vi "ImportBitmap2.vi"(8 "error in (no error)":errorcluster) -> (0 "error out":errorcluster, 1 "color table":u32[](array[colorbox]), 2 "pixmap data":u8[](array[numeric]), 3 "rect":T1, 5 "bit depth(8)":i32=8)   [LabVIEW 2013, in "main.lvlib"]
uses:
  main.lvlib
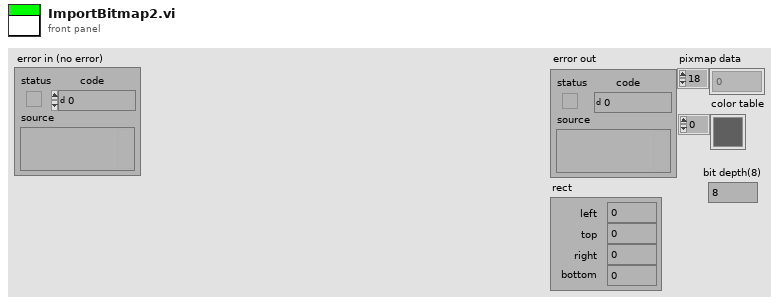
[diagram p1: front panel]
types:
  T1 = cluster{"left":i16, "top":i16, "right":i16, "bottom":i16}
  T2 = typedef "CLIP Refnum.ctl" = refnum<k1>
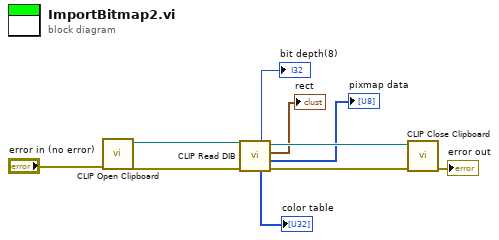
[diagram p0: block diagram]
diagram:
  n1 = call "CLIP Open Clipboard.vi"("error in (no error)"="error in (no error)") -> ("error out"=w9:errorcluster, "clipboard ref"=w10:T2)  [unwired: 5 in]
  n2 = call "CLIP Read DIB.vi"("error in (no error)"=w9, "clipboard ref"=w10) -> ("error out"=w6:errorcluster, "pixmap data"=→"pixmap data":u8[], "rect"=→"rect":T1, "clipboard ref out"=w5:T2, "color table"=→"color table":u32[], "bit depth(8)"=→"bit depth(8)":i32)  [unwired: 4 in]
  n3 = call "CLIP Close Clipboard.vi"("error in (no error)"=w6, "clipboard ref"=w5) -> ("error out"=→"error out":errorcluster)  [unwired: 5 in]
